vi "Read Kamikaze DVR.vi"(8 "error in (no error)":errorcluster, 11 "Mother in":refnum<class "Mother.lvclass">) -> (0 "error out":errorcluster, 2 "Kamikaze DVR":T1, 3 "Mother out":refnum<class "Mother.lvclass">)   [LabVIEW 2014, in "Mother.lvclass"]
uses:
  Mother.lvclass
  Kamikaze DVR.ctl
  Mother.lvclass/Mother.ctl
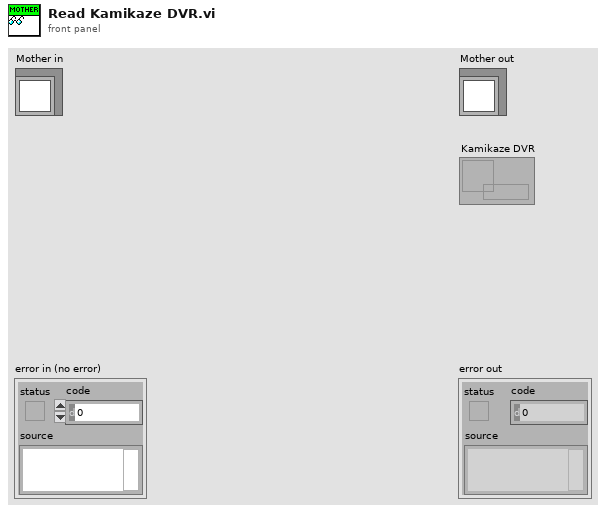
[diagram p1: front panel]
types:
  T1 = typedef "Mother.lvclass/Kamikaze DVR.ctl" = refnum<data-value>
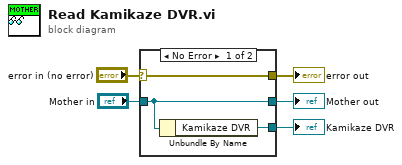
[diagram p0: block diagram]
diagram:
  n1 = case shown="No Error" "error in (no error)" {
    selector: "error in (no error)" -> [w8 w9]
    tunnel: [w8 w9] -> w4
    tunnel: [w7 w10] -> w2
    tunnel: "Mother in" -> [w7 w10]
    tunnel: [w6 _] -> w1
    frame No Error {
      n2 = Unbundle By Name(w7) -> ("Kamikaze DVR"=w6:T1)
    }
    frame Error {
    }
  }
  "error out" <- w4
  "Mother out" <- w2
  "Kamikaze DVR" <- w1
